vi "Resolver Calibration Test Bench.vi"() -> ()   [LabVIEW 2014]
uses:
  <vilib>/Platform/TimedLoop/XDataNode/XDataNode.xnode
  <vilib>/Platform/TimedLoop/XDataNode/nitl_modes.ctl
  <vilib>/Platform/TimedLoop/XDataNode/XDNodeRunTimeDep.lvlib
  <vilib>/Platform/TimedLoop/XDataNode/wakeup.ctl
  <vilib>/Platform/TimedLoop/XDataNode/timing_clust.ctl
  Global Data.vi
  AIR Status.ctl
panel:
  in  "Spindown":bool
  in  "Requested Torque (Nm)":dbl format="%#_13g"
  in  "CAN Offset":u32=512 format="%x"
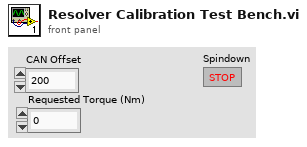
[diagram p1: front panel]
types:
  T1 = typedef "AIR Status.ctl" = enum16{"Off", "Precharge", "On"}
  T2 = typedef "XDNodeRunTimeDep.lvlib/timing_clust.ctl" = cluster{"Expected End [f-1]":u64, "Actual End [f-1]":u64, "Finished Late? [f-1]":bool, "Expected End [i-1]":u64, "Actual End [i-1]":u64, "Finished Late? [i-1]":bool, "Expected Start [i]":u64, "Actual Start [i]":u64, "Expected Start [f]":u64, "Actual Start [f]":u64, "Source Name":string, "Structure Name":string, "Period":i64, "Deadline":i64, "Offset":i64, "Start":i64, "Priority":i32, "Timeout":i32, "Mode":T3, "Wakeup Reason":T4, "Error":errorcluster, "Source Type":string, "Secondary Source Type":string, "Global End Time":u64, "Global Start Time":u64, "Frame Duration":u64, "Iteration Duration":u64, "Assigned CPU":i32, "I/O Scan Engine Mode":u32}
  T3 = typedef "XDNodeRunTimeDep.lvlib/nitl_modes.ctl" = enum32{"No Change", "Process missed periods, maintain original phase", "Discard missed periods, maintain original phase", "Process missed periods, ignore original phase", "Discard missed periods, ignore original phase"}
  T4 = typedef "XDNodeRunTimeDep.lvlib/wakeup.ctl" = enum32{"Normal", "Aborted", "Asynchronous wakeup", "Timing source error", "Timed loop error", "Timeout"}
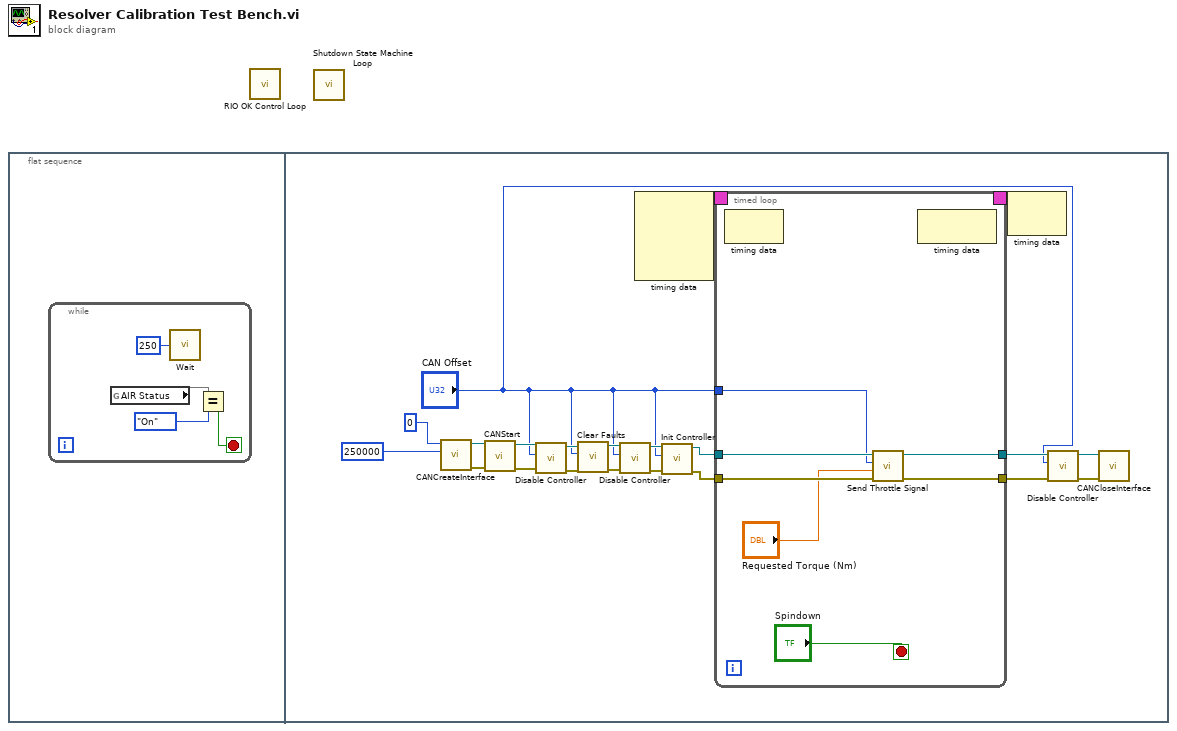
[diagram p0: block diagram]
diagram:
  n1 = flat-sequence {
    frame #0 {
      n2 = while {
        stop <- w2 stop-if-true
        n3 = global read "Global Data.vi" "AIR Status"() -> (w4)
        n4 = call "Wait"("Count(mSec)"=u32 250) -> ()  [unwired: 1 out]
        n5 = Equal?(x=w4, y=AIR_Status."On") -> (x = y?=w2:bool)
      }
    }
    frame #1 {
      n6 = call <vilib>:"CANCreateInterface.vi"("baud rate (125000 bps)"=u32 250000, "interface index"=u32 0) -> ("error out"=w21:errorcluster, "interface object out"=w20:refnum<k20>)  [unwired: 8 in]
      n7 = call <vilib>:"CANStart.vi"("error in (no error)"=w21, "interface object in"=w20) -> ("error out"=w18:errorcluster, "interface object out"=w19:refnum<k20>)  [unwired: 8 in]
      n8 = call "Disable Controller.vi"("error in (no error)"=w18, "CAN Offset"="CAN Offset", "interface object in"=w19) -> ("error out"=w6:errorcluster, "interface object out"=w7:refnum<k20>)  [unwired: 7 in]
      n9 = call "Clear Faults.vi"("error in (no error)"=w6, "CAN Offset"="CAN Offset", "interface object in"=w7) -> ("error out"=w8:errorcluster, "interface object out"=w9:refnum<k20>)  [unwired: 7 in]
      n10 = call "Disable Controller.vi"("error in (no error)"=w8, "CAN Offset"="CAN Offset", "interface object in"=w9) -> ("error out"=w10:errorcluster, "interface object out"=w11:refnum<k20>)  [unwired: 7 in]
      n11 = node-c288() -> (w25:T2)  [unwired: 4 in]
      n12 = call "Init Controller.vi"("error in (no error)"=w10, "CAN Offset"="CAN Offset", "interface object in"=w11) -> ("error out"=w16:errorcluster, "interface object out"=w17:refnum<k20>)  [unwired: 7 in]
      n13 = timed-loop {
        timing: w25 -> [_]
        timing-out: [_] -> w24
        tunnel: w17 -> [w32]
        tunnel: w16 -> [w31]
        tunnel: "CAN Offset" -> [w30]
        tunnel: [w27] -> w15
        tunnel: [w26] -> w14
        stop <- "Spindown" stop-if-true
        n14 = node-c288() -> ()  [unwired: 1 in, 1 out]
        n15 = call "Send Throttle Signal.vi"("error in (no error)"=w31, "Requested Torque (Nm)"="Requested Torque (Nm)", "CAN Offset"=w30, "interface object in"=w32) -> ("error out"=w26:errorcluster, "interface object out"=w27:refnum<k20>)  [unwired: 6 in]
        n16 = node-c288() -> ()  [unwired: 1 in, 1 out]
      }
      n17 = node-c288(w24) -> ()  [unwired: 1 out]
      n18 = call "Disable Controller.vi"("error in (no error)"=w14, "CAN Offset"="CAN Offset", "interface object in"=w15) -> ("error out"=w13:errorcluster, "interface object out"=w12:refnum<k20>)  [unwired: 7 in]
      n19 = call <vilib>:"CANCloseInterface.vi"("error in (no error)"=w13, "interface object in"=w12) -> ()  [unwired: 9 in, 1 out]
    }
  }
  n20 = call "RIO OK Control Loop.vi"() -> ()  [unwired: 12 in]
  n21 = call "Shutdown State Machine Loop.vi"() -> ()  [unwired: 12 in]
